vi "Enable or Disable UI.vi"(7 "Action":T1(ring), 8 "Error In":errorcluster, 11 "Control Refs":refnum<vi>[](array[refnum])) -> (0 "Error Out":errorcluster)   [LabVIEW 2017]
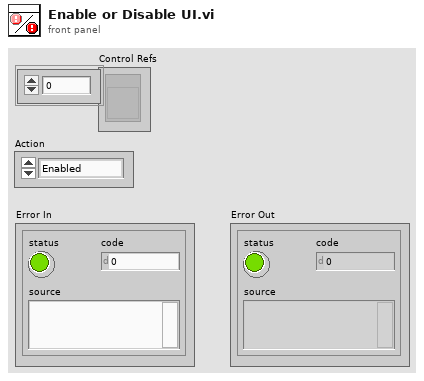
[diagram p1: front panel]
types:
  T1 = enum8{"Enabled", "Disabled", "Disabled and Grayed Out"}
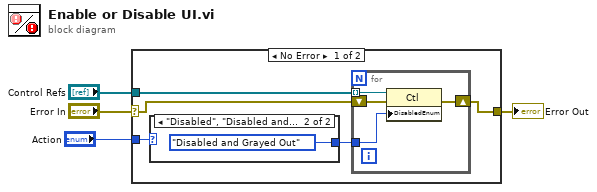
[diagram p0: block diagram]
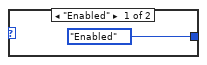
[diagram p2: hidden frame]
diagram:
  n1 = case shown="No Error" "Error In" {
    selector: "Error In" -> [w6 w16]
    tunnel: [w5 w16] -> w3
    tunnel: "Control Refs" -> [w9 _]
    tunnel: "Action" -> [w8 _]
    frame No Error {
      n2 = case shown="\"Disabled\", \"Disabled and Grayed Out\"" w8 {
        tunnel: [T1."Enabled" ("Disabled") T1."Disabled and Grayed Out" ("Disabled")] -> w7
        frame "Enabled" {
        }
        frame "Disabled", "Disabled and Grayed Out" {
        }
      }
      n3 = for {
        tunnel: w9 -> [w15] mode=indexing
        tunnel: w7 -> [w14]
        shift-right: [w12] -> w5
        shift-left: w6 -> [w13]
        n4 = property class="Ctl"(reference=w15, error in=w13, "DisabledEnum"=w14) -> (error out=w12:errorcluster)  [unwired: 1 out]
      }
    }
    frame Error {
    }
  }
  "Error Out" <- w3
